vi "DSF.Engine.Builder.Set ID.vi"(10 "ID":i32, 11 "Builder in":refnum<class "DSF.Engine.Builder.lvclass">) -> (3 "Builder out":refnum<class "DSF.Engine.Builder.lvclass">)   [LabVIEW 2016, in "DSF.Engine.lvlib" / "DSF.Engine.Builder.lvclass"]
uses:
  DSF.Engine.Builder.lvclass
  DSF.Engine.Builder.lvclass/DSF.Engine.Builder.ctl
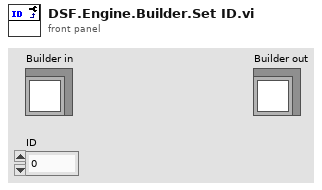
[diagram p1: front panel]
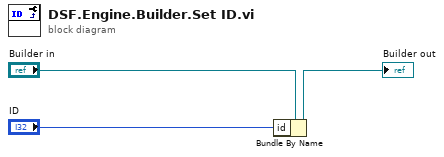
[diagram p0: block diagram]
diagram:
  n1 = Bundle By Name(cluster="Builder in", "id"="ID") -> (→"Builder out":refnum<class "DSF.Engine.Builder.lvclass">)
